vi "(SUBVI) - Drop Off.vi"(10 "Motors":T2=7 items=["Port A", "Port B", "Port C", "Port D"], 11 "NXT/EV3":T1) -> (3 "NXT/EV3 2":T1)   [LabVIEW 2016]
uses:
  <vilib>/NXT/Subs/LVHSConnector.ctl
  <vilib>/NXT/LegoClasses/BrickReference/BrickReference.lvclass
  <vilib>/NXT/Block Support/NXT_OutputPort.ctl
  testrobot.lvrbt
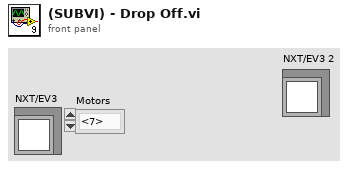
[diagram p1: front panel]
types:
  T1 = typedef "LVHSConnector.ctl" = refnum<class "BrickReference.lvclass">
  T2 = typedef "NXT_OutputPort.ctl" = u8
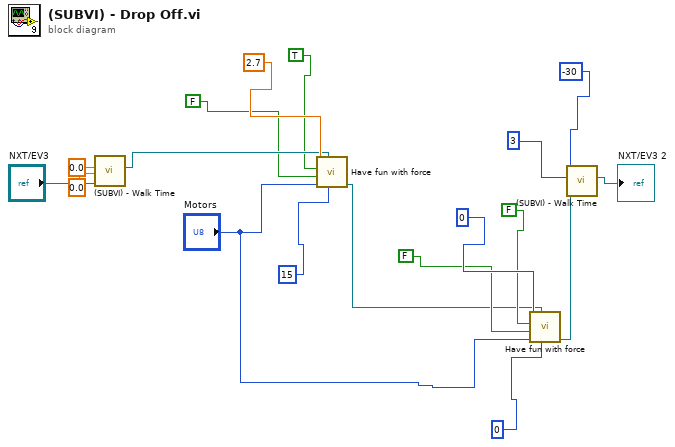
[diagram p0: block diagram]
diagram:
  n1 = call "(SUBVI) - Walk Time.vi"("NXT/EV3"="NXT/EV3", "Time walking"=0.0, "Walk Speed"=0.0) -> ("NXT/EV3 2"=w13:T1)  [unwired: 8 in]
  n2 = call "Have fun with force.vi"("Speed"=15, "NXT/EV3"=w13, "Motors"="Motors", "Up/Down"=FALSE, "Run"=TRUE, "Time"=2.7) -> ("NXT/EV3 2"=w3:T1)  [unwired: 5 in]
  n3 = call "Have fun with force.vi"("Speed"=0, "NXT/EV3"=w3, "Motors"="Motors", "Up/Down"=FALSE, "Run"=FALSE, "Time"=0) -> ("NXT/EV3 2"=w2:T1)  [unwired: 5 in]
  n4 = call "(SUBVI) - Walk Time.vi"("NXT/EV3"=w2, "Time walking"=3, "Walk Speed"=-30) -> ("NXT/EV3 2"=→"NXT/EV3 2":T1)  [unwired: 8 in]
